vi "subDFD_Narrowband Filtering Specs Conversion.vi"(8 "center freq":dbl, 9 "stopband":dbl, 10 "passband":dbl, 11 "filter type":T2(ring)) -> (3 "freq specs [Hz]":T1={"fpass 1"=0.015, "fstop 1"=0.02, "fpass 2 "=0.0, "fstop 2"=0.0})   [LabVIEW 2020]
uses:
  <vilib>/addons/Digital Filter Design/_Objects.llb/DFD Filter Frequence Specification (Design).ctl
  <vilib>/addons/Digital Filter Design/NI_DigFilterLicensed.lvlib
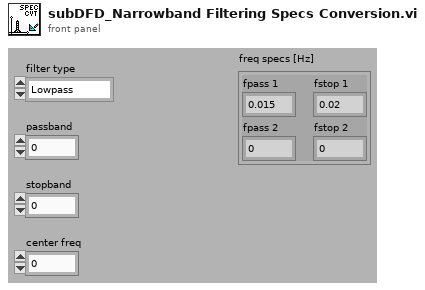
[diagram p1: front panel]
types:
  T1 = typedef "NI_DigFilterLicensed.lvlib/DFD Filter Frequence Specification (Design).ctl" = cluster{"fpass 1":dbl, "fstop 1":dbl, "fpass 2 ":dbl, "fstop 2":dbl}
  T2 = enum32{"Lowpass", "Highpass", "Bandpass", "Bandstop"}
  T3 = cluster{"passband":dbl, "stopband":dbl, dbl, dbl}
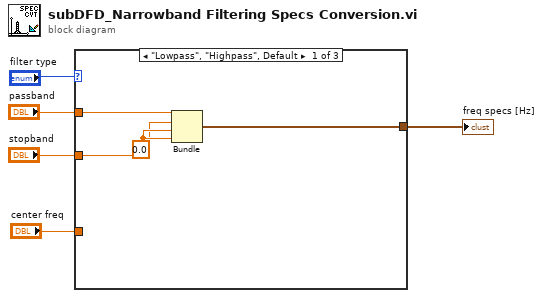
[diagram p0: block diagram]
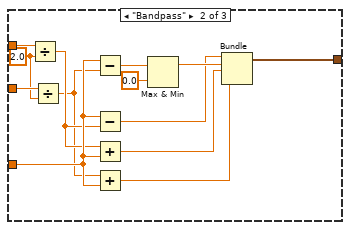
[diagram p2: hidden frame]
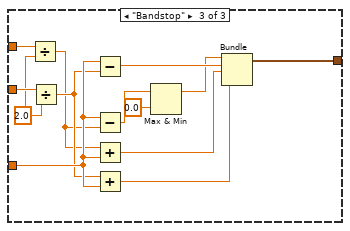
[diagram p3: hidden frame]
diagram:
  n1 = case shown="\"Lowpass\", \"Highpass\", Default" "filter type" {
    tunnel: "passband" -> [w8 w13 w34]
    tunnel: "stopband" -> [w7 w11 w32]
    tunnel: [w6 w15 w29] -> w1
    tunnel: "center freq" -> [_ w18 w33]
    frame "Lowpass", "Highpass", Default {
      w9 = 0.0
      n2 = Bundle("passband"=w8, "stopband"=w7, w9, w9) -> (w6:T3)  [unwired: 1 out]
    }
    frame "Bandpass" {
      w10 = 2.0 ("y")
      n3 = Divide(x=w13, y=w10) -> (x/y=w14:dbl)
      n4 = Divide(x=w11, y=w10) -> (x/y=w12:dbl)
      n5 = Subtract(x=w18, y=w12) -> (x-y=w22:dbl)
      n6 = Subtract(x=w18, y=w14) -> (x-y=w19:dbl)
      n7 = Add(x=w14, y=w18) -> (x+y=w16:dbl)
      n8 = Add(x=w12, y=w18) -> (x+y=w17:dbl)
      n9 = Max & Min(x=w22, y=0.0) -> (max(x,y)=w20:dbl)  [unwired: 1 out]
      n10 = Bundle(w19, w20, w16, w17) -> (w15:cluster{dbl, dbl, dbl, dbl})  [unwired: 1 out]
    }
    frame "Bandstop" {
      w23 = 2.0 ("y")
      n11 = Divide(x=w34, y=w23) -> (x/y=w24:dbl)
      n12 = Divide(x=w32, y=w23) -> (x/y=w25:dbl)
      n13 = Subtract(x=w33, y=w25) -> (x-y=w28:dbl)
      n14 = Subtract(x=w33, y=w24) -> (x-y=w27:dbl)
      n15 = Add(x=w24, y=w33) -> (x+y=w30:dbl)
      n16 = Add(x=w25, y=w33) -> (x+y=w31:dbl)
      n17 = Max & Min(x=w27, y=0.0) -> (max(x,y)=w26:dbl)  [unwired: 1 out]
      n18 = Bundle(w26, w28, w30, w31) -> (w29:cluster{dbl, dbl, dbl, dbl})  [unwired: 1 out]
    }
  }
  "freq specs [Hz]" <- w1
